vi "Query Rels Ready.vi"(8 "Error In (no error)":errorcluster, 9 "Value Type (0: XY)":u16(ring) items=["XY", "R[dBm] Phi"], 10 "Scan Point (1)":i32=1, 11 "VISA Resource Name":refnum<visa-resource-name>) -> (0 "Error Out":errorcluster, 2 "Rel Values Status":bool, 3 "VISA Resource Name Out":refnum<visa-resource-name>)   [LabVIEW 2010, in "Stanford Research 844.lvlib"]
doc: "This VI queries whether any Rel Values are stored for the current frequency."
uses:
  <instrlib>/Stanford Research 844/Stanford Research 844.lvlib
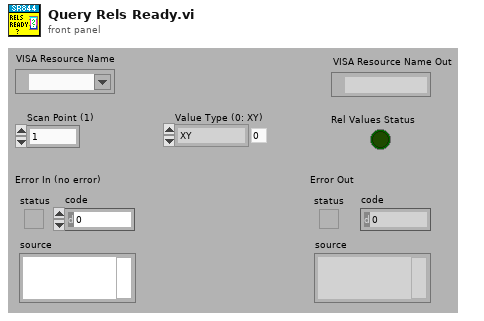
[diagram p1: front panel]
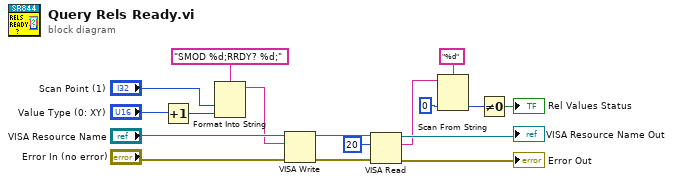
[diagram p0: block diagram]
diagram:
  n1 = Increment(x="Value Type (0: XY)") -> (x+1=w2:u16)
  n2 = Format Into String(format string="SMOD %d;RRDY? %d;", "Scan Point (1)", w2) -> (resulting string=w1:string)  [unwired: 2 in, 1 out]
  n3 = VISA Write(VISA resource name="VISA Resource Name", write buffer=w1, error in (no error)="Error In (no error)") -> (VISA resource name out=w12:refnum<visa-resource-name>, error out=w13:errorcluster)  [unwired: 1 out]
  n4 = VISA Read(VISA resource name=w12, byte count=u32 20 ("byte count (0)"), error in (no error)=w13) -> (VISA resource name out=→"VISA Resource Name Out":refnum<visa-resource-name>, read buffer=w6:string, error out=→"Error Out":errorcluster)  [unwired: 1 out]
  n5 = Scan From String(format string="%d", input string=w6, default 1=0 ("default value 1")) -> (output 1=w5:i32)  [unwired: 2 in, 3 out]
  n6 = Not Equal To 0?(x=w5) -> (x != 0?=→"Rel Values Status":bool)
